vi "Scheduler.vi"(8 "error in":errorcluster, 10 "Safe State on Engine Error?":bool=TRUE, 11 "Module Info In":T2) -> (0 "error out":errorcluster, 2 "Safe State?":bool, 3 "Module Info Out":T2)   [LabVIEW 2013, in "Standard Engine Runtime.lvclass"]
uses:
  Standard Engine Runtime.lvclass
  Module Execution Info.ctl
  <vilib>/NI/Tag Bus Module Framework/runtime/TBM module execution interface.lvclass
  Data Table with Transfer Spec.ctl
  <vilib>/NI/Tag Bus/table/data table.ctl
  <vilib>/NI/Tag Bus/table/transfer specification.ctl
  <vilib>/NI/Tag Bus/tag/Data Type.ctl
  Configuration/Module Decimation.ctl
  Configuration/Module Error Configuration.ctl
  Configuration/Error Actions By Category.ctl
  <vilib>/NI/Tag Bus Module Framework/runtime/error classification.ctl
  Configuration/Error Actions.ctl
  Error Queue.ctl
  Delete Module Index.vi
  <vilib>/NI/Tag Bus/tag/tag descriptor.lvclass
  Configuration/Standard Engine Configuration.lvclass
  <vilib>/NI/Tag Bus/table/data table.lvlib
panel:
  in  "Error Queue":T1
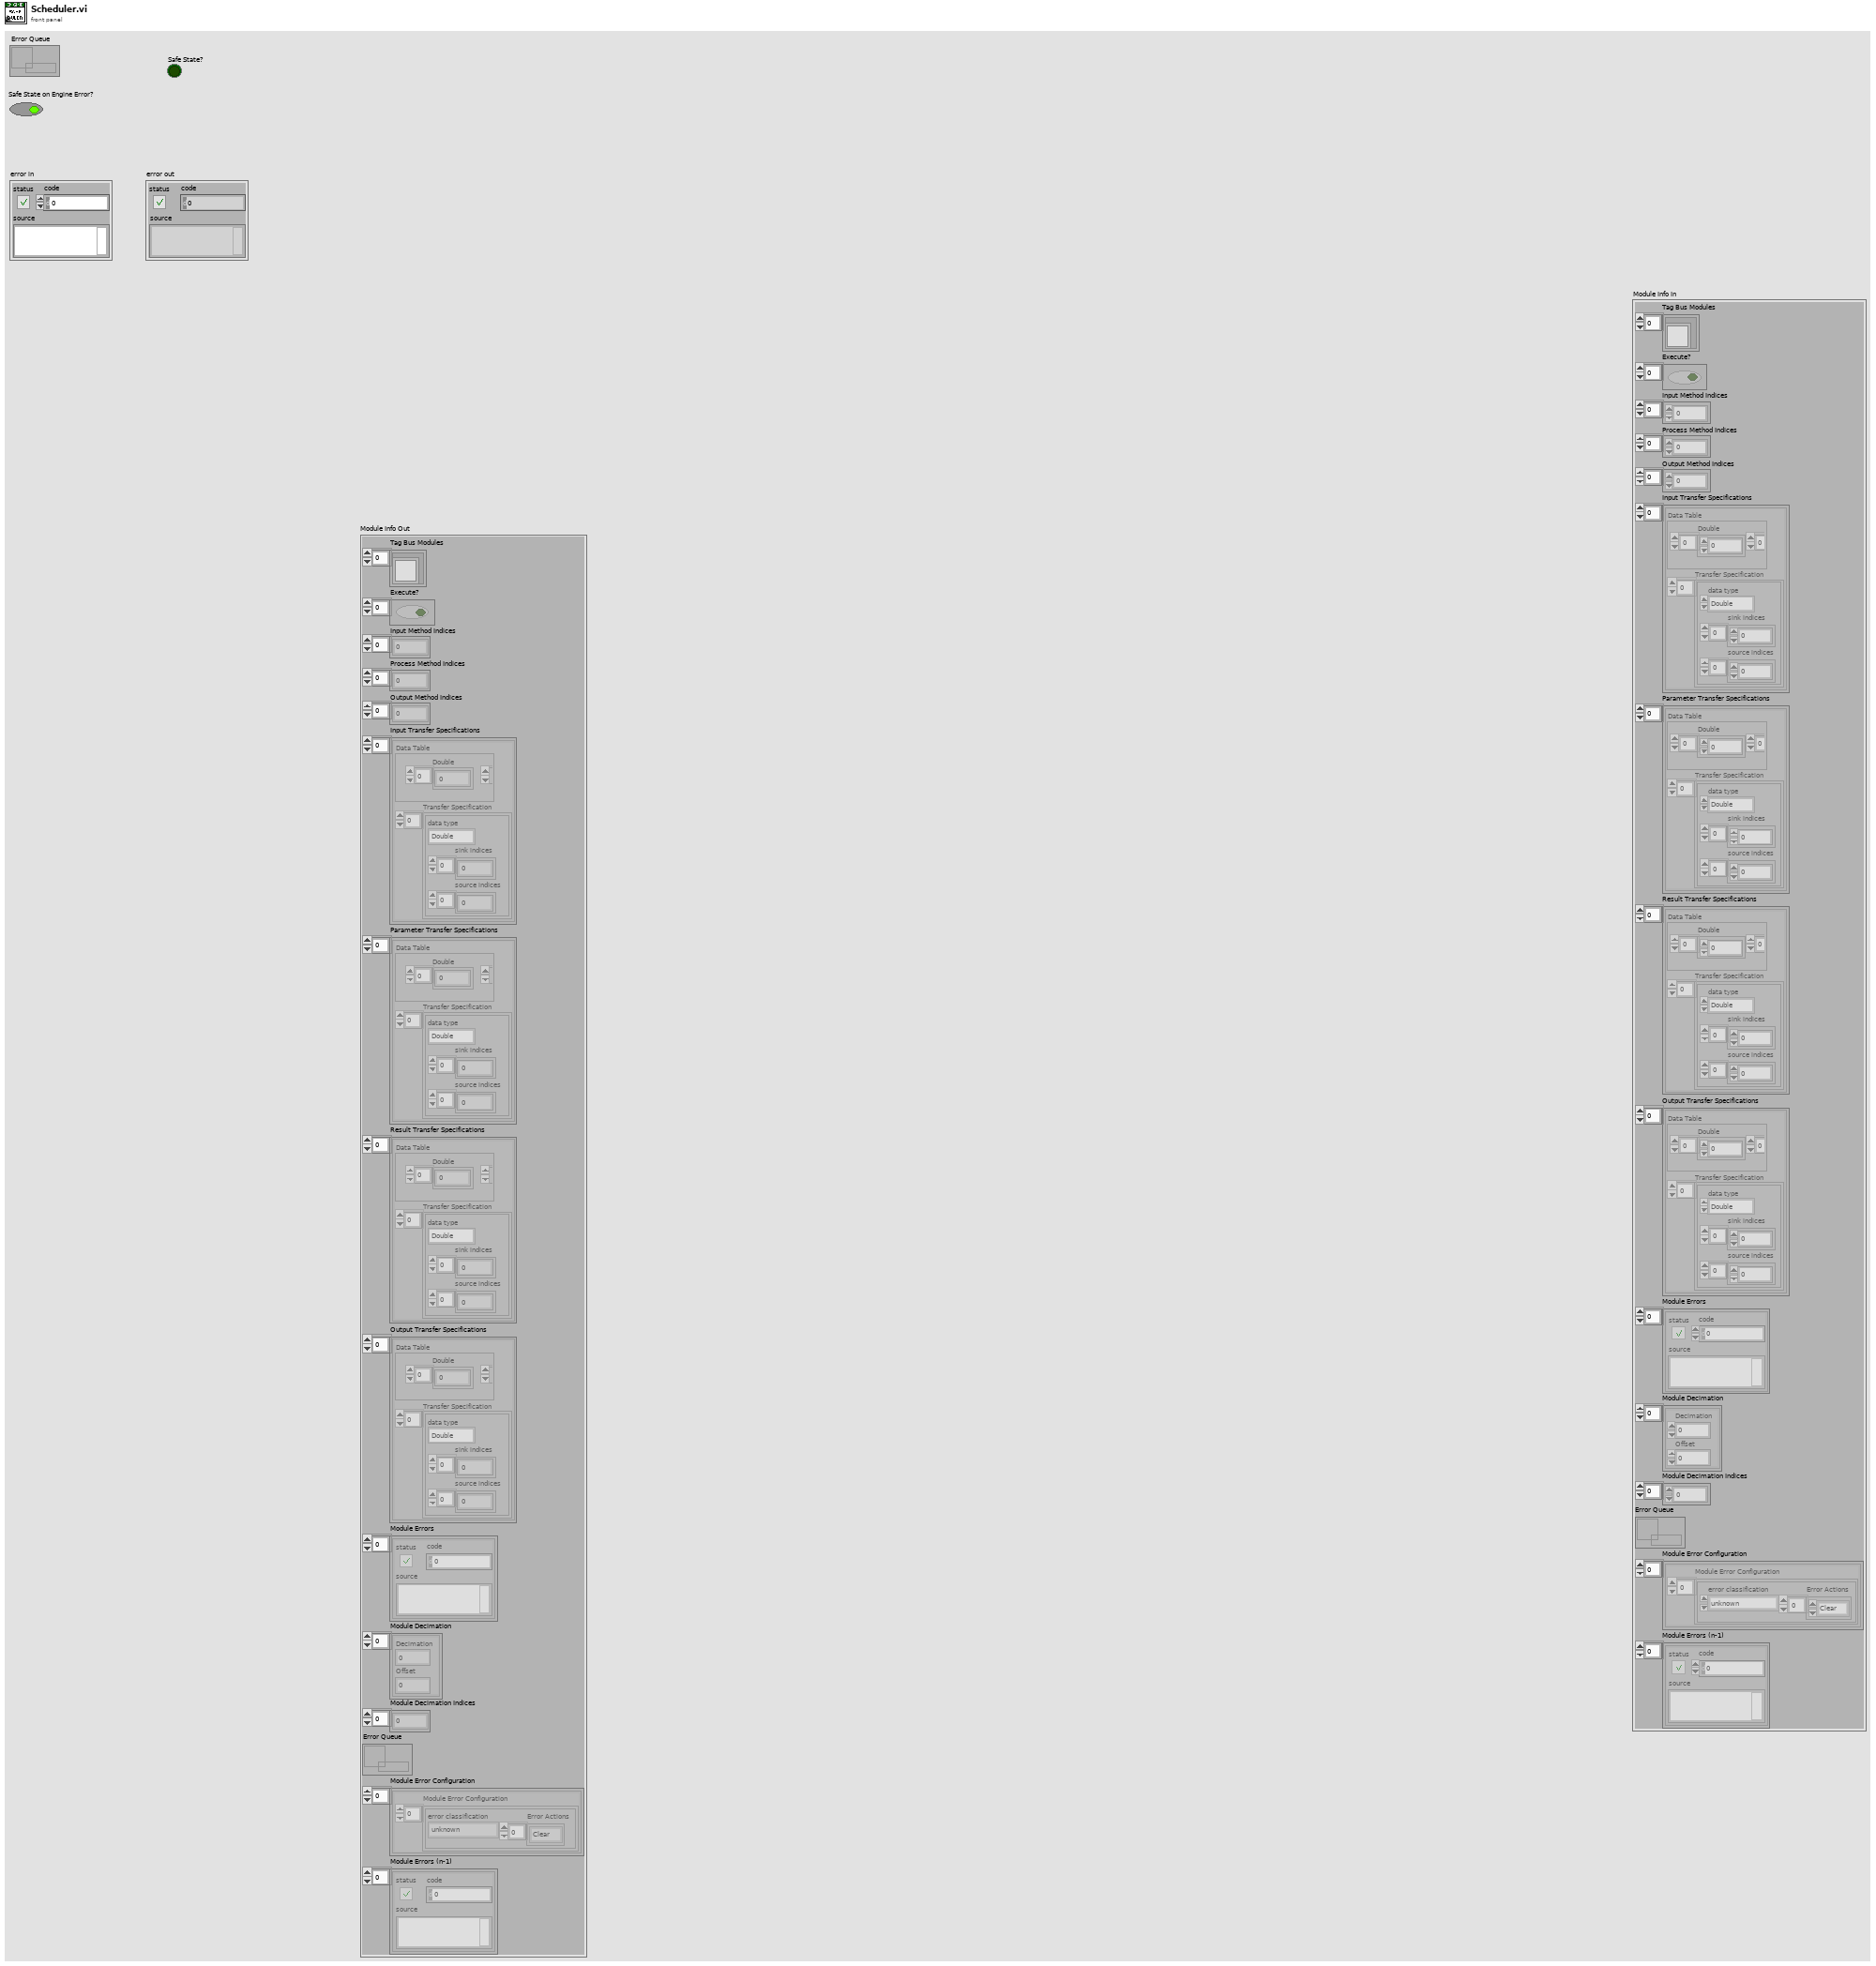
[diagram p1: front panel]
types:
  T1 = typedef "Standard Engine Runtime.lvclass/Error Queue.ctl" = refnum<queue>
  T2 = typedef "Standard Engine Runtime.lvclass/Module Execution Info.ctl" = cluster{"Tag Bus Modules":refnum<class "TBM module execution interface.lvclass">[], "Execute?":bool[], "Input Method Indices":i32[], "Process Method Indices":i32[], "Output Method Indices":i32[], "Input Transfer Specifications":T3[], "Parameter Transfer Specifications":T3[], "Result Transfer Specifications":T3[], "Output Transfer Specifications":T3[], "Module Errors":errorcluster[], "Module Decimation":T7[], "Module Decimation Indices":i32[], "Error Queue":refnum<queue>, "Module Error Configuration":T8[], "Module Errors (n-1)":errorcluster[]}
  T3 = typedef "Standard Engine Runtime.lvclass/Data Table with Transfer Spec.ctl" = cluster{"Data Table":T4, "Transfer Specification":T5[]}
  T4 = typedef "tag bus.lvlib/data table.lvlib/data table.ctl" = cluster{"Double":dbl[], "Single":sgl[], "I64":i64[], "I32":i32[], "I16":i16[], "I8":i8[], "U64":u64[], "U32":u32[], "U16":u16[], "U8":u8[], "Boolean":bool[], "String":string[], "Array of Double":cluster{"DBL Array":dbl[]}[], "Array of Single":cluster{"SGL Array":sgl[]}[], "Array of I64":cluster{"I64 Array":i64[]}[], "Array of I32":cluster{"I32 Array":i32[]}[], "Array of I16":cluster{"I16 Array":i16[]}[], "Array of I8":cluster{"I8 Array":i8[]}[], "Array of U64":cluster{"U64 Array":u64[]}[], "Array of U32":cluster{"U32 Array":u32[]}[], "Array of U16":cluster{"U16 Array":u16[]}[], "Array of U8":cluster{"U8 Array":u8[]}[], "Array of Boolean":cluster{"Boolean Array":bool[]}[], "Array of String":cluster{"String Array":string[]}[]}
  T5 = typedef "tag bus.lvlib/data table.lvlib/transfer specification.ctl" = cluster{"data type":T6, "sink indices":i32[], "source indices":i32[]}
  T6 = typedef "tag bus.lvlib/tag descriptor.lvclass/Data Type.ctl" = enum16{"Double", "Single", "I64", "I32", "I16", "I8", "U64", "U32", "U16", "U8", "Boolean", "String", "Array of Double", "Array of Single", "Array of I64", "Array of I32", "Array of I16", "Array of I8", "Array of U64", "Array of U32", "Array of U16", "Array of U8", "Array of Boolean", "Array of String"}
  T7 = typedef "Standard Engine Configuration.lvclass/Module Decimation.ctl" = cluster{"Decimation":u16, "Offset":u16}
  T8 = typedef "Standard Engine Configuration.lvclass/Module Error Configuration.ctl" = cluster{"Module Error Configuration":T9[]}
  T9 = typedef "Standard Engine Configuration.lvclass/Error Actions By Category.ctl" = cluster{"error classification":T10, "Error Actions":T11[]}
  T10 = typedef "TBM module execution interface.lvclass/error classification.ctl" = enum16{"unknown", "none", "trivial", "recoverable", "critical"}
  T11 = typedef "Standard Engine Configuration.lvclass/Error Actions.ctl" = enum16{"Clear", "Notify", "Stop Component", "Stop Engine", "Safe State", "Attempt Recovery"}
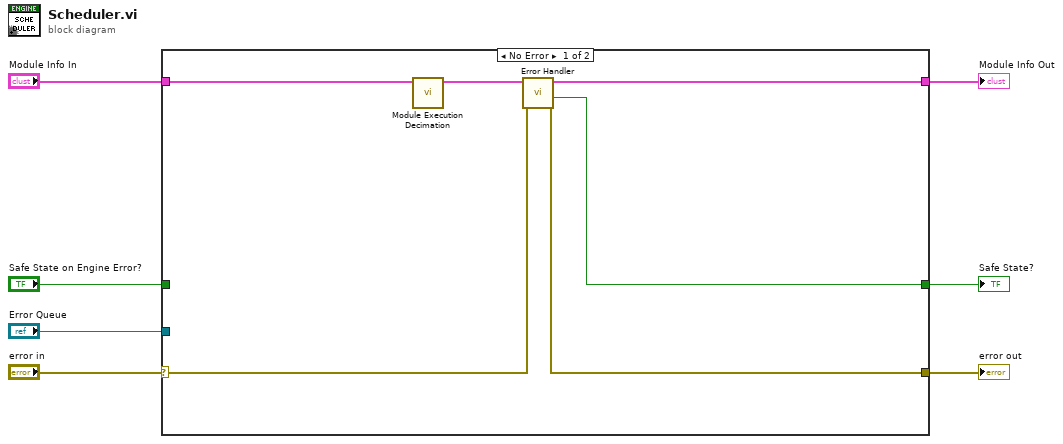
[diagram p0: block diagram]
diagram:
  n1 = case shown="No Error" "error in" {
    selector: "error in" -> [w13 w16]
    tunnel: "Module Info In" -> [w11 w15]
    tunnel: [w9 w15] -> w6
    tunnel: [w8 w16] -> w5
    tunnel: "Safe State on Engine Error?" -> [_ w14]
    tunnel: [w12 w14] -> w1
    tunnel: "Error Queue" -> [_ _]
    frame No Error {
      n2 = call "Module Execution Decimation.vi"("Module Info In"=w11) -> ("Module Info Out"=w10:T2)  [unwired: 10 in]
      n3 = call "Error Handler.vi"("Engine Error"=w13, "Component Info In"=w10) -> ("Engine Errors"=w8:errorcluster, "Safe State"=w12:bool, "Component Info Out"=w9:T2)  [unwired: 7 in]
    }
    frame Error {
    }
  }
  "Module Info Out" <- w6
  "error out" <- w5
  "Safe State?" <- w1
